vi "DCTMeasure.vi"(1 "Duration Time":refnum<vi>, 2 "Update Time":refnum<vi>, 3 "Time Left":refnum<vi>, 7 "Detectors Select":enum32{"4 Detectors", "8 Detectors"}(ring), 12 "Detector Buttons":refnum<vi>, 13 "Detector Indicators":refnum<vi>, 14 "g2":refnum<vi>) -> (6 "Intensity data":string, 8 "tau data":string, 10 "g2 data":string)   [LabVIEW 2011]
uses:
  DCS/flex05-4chPascal.dll
  DCS/flex05oem8chautoPASCAL.dll
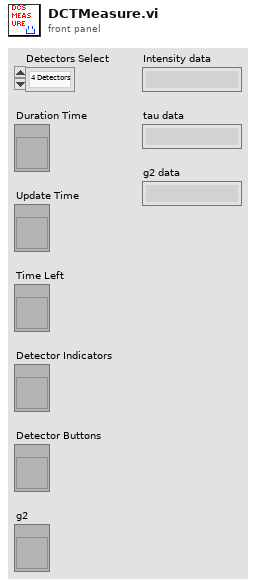
[diagram p1: front panel]
types:
  T1 = cluster{"btnDet 1":bool, "btnDet 2":bool, "btnDet 3":bool, "btnDet 4":bool, "btnDet 5":bool, "btnDet 6":bool, "btnDet 7":bool, "btnDet 8":bool}
  T2 = cluster{"Intensity Array[0]":sgl, "Intensity Array[1]":sgl, "Intensity Array[2]":sgl, "Intensity Array[3]":sgl, "Intensity Array[4]":sgl, "Intensity Array[5]":sgl, "Intensity Array[6]":sgl, "Intensity Array[7]":sgl}
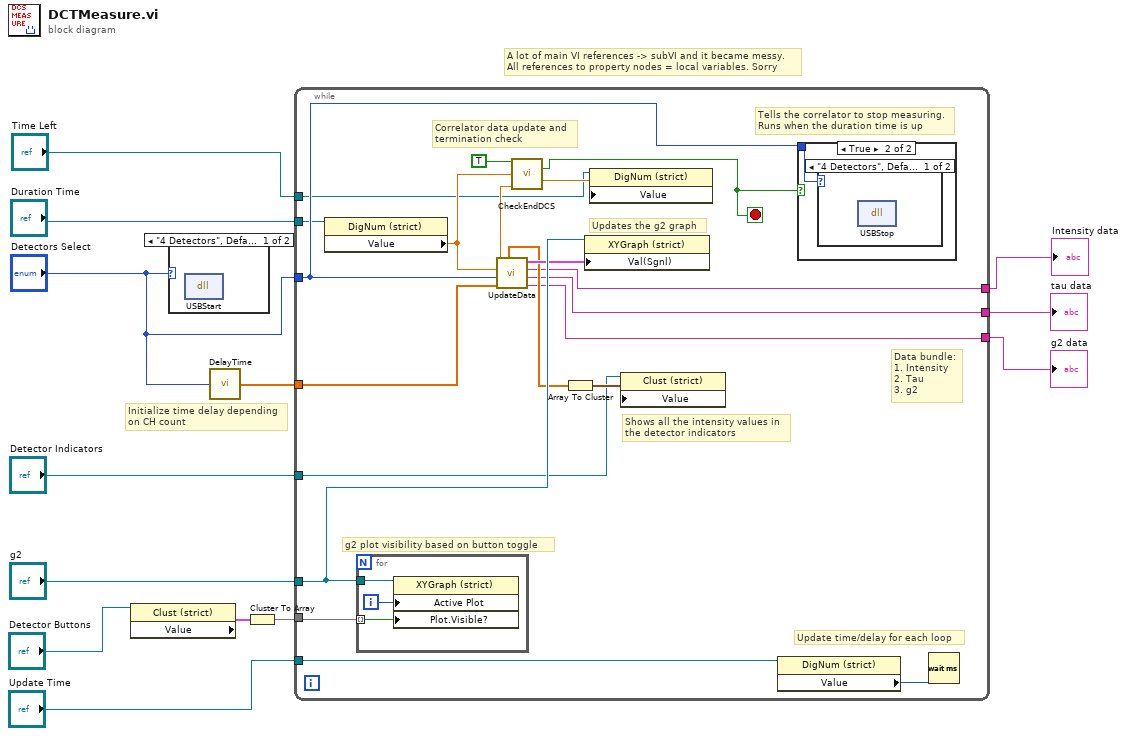
[diagram p0: block diagram]
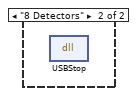
[diagram p3: hidden frame]
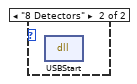
[diagram p4: hidden frame]
diagram:
  # "A lot of main VI references -> subVI and it became messy.\nAll references to property nodes = local variables. Sorry"
  # "Initialize time delay depending\non CH count"
  n1 = property class="Clust (strict)"(reference="Detector Buttons") -> ("Value"=w7:T1)  [unwired: 1 in, 2 out]
  n2 = case shown="\"4 Detectors\", Default" "Detectors Select" {
    frame "4 Detectors", Default {
      n3 = dll-call lib="C:/LABVIEWcodesWorksInC/UnderDeveopmentNeedChecking/Vincent2017/Dependencies/DCS/flex05-4chPascal.dll" fn="USBStart" label="CH4: USBStart"() -> ()  [unwired: 4 in, 2 out]
    }
    frame "8 Detectors" {
      n4 = dll-call lib="C:/LABVIEWcodesWorksInC/UnderDeveopmentNeedChecking/Vincent2017/Dependencies/DCS/flex05oem8chautoPASCAL.dll" fn="USBStart" label="CH8: USBStart"() -> ()  [unwired: 4 in, 2 out]
    }
  }
  n5 = call "DelayTime.vi"("Detector Select"="Detectors Select") -> ("Delaytime"=w6:sgl[])
  n6 = Cluster To Array(cluster=w7) -> (array=w8:bool[])
  n7 = while {
    tunnel: "Detectors Select" -> [w18]
    tunnel: w6 -> [w25]
    tunnel: w8 -> [w33]
    tunnel: "g2" -> [w27]
    tunnel: [w21] -> w11
    tunnel: [w20] -> w12
    tunnel: [w19] -> w13
    tunnel: "Update Time" -> [w17]
    tunnel: "Duration Time" -> [w16]
    tunnel: "Time Left" -> [w15]
    tunnel: "Detector Indicators" -> [w14]
    stop <- w22 stop-if-true
    # "Data bundle:\n1. Intensity\n2. Tau\n3. g2"
    # "Correlator data update and\ntermination check"
    # "Updates the g2 graph"
    # "Shows all the intensity values in\nthe detector indicators"
    # "Update time/delay for each loop"
    # "g2 plot visibility based on button toggle"
    # "Tells the correlator to stop measuring.\nRuns when the duration time is up"
    n8 = property class="DigNum (strict)"(reference=w16) -> ("Value"=w31:sgl)  [unwired: 1 in, 2 out]
    n9 = for {
      tunnel: w33 -> [w36] mode=indexing
      tunnel: w27 -> [w37]
      i -> [w35]
      n10 = property on="Property Node" class="XYGraph (strict)"(reference=w37, "Active Plot"=w35, "Plot.Visible?"=w36) -> ()  [unwired: 1 in, 2 out]
    }
    n11 = call "UpdateData.vi"("Delay Time"=w25, "Detector Select"=w18, "Duration Time (ms)"=w31) -> ("g2 data"=w19:string, "tau data"=w20:string, "Intensity data"=w21:string, "g2 Display"=w26:cluster{"Delay Time":sgl[], sgl[]}[], "Intensity Array"=w23:sgl[], "Elapsed Time(s)"=w28:sgl)  [unwired: 1 out]
    n12 = call "CheckEndDCS.vi"("start"=TRUE, "duration time"=w31, "elapsed time"=w28) -> ("stopped"=w22:bool, "time left"=w30:sgl)  [unwired: 11 in]
    n13 = Array To Cluster(array=w23) -> (cluster=w24:T2)
    n14 = property class="XYGraph (strict)"(reference=w27, "Val(Sgnl)"=w26) -> ()  [unwired: 1 in, 2 out]
    n15 = property class="DigNum (strict)"(reference=w15, "Value"=w30) -> ()  [unwired: 1 in, 2 out]
    n16 = property class="Clust (strict)"(reference=w14, "Value"=w24) -> ()  [unwired: 1 in, 2 out]
    n17 = property class="DigNum (strict)"(reference=w17) -> ("Value"=w32:u32)  [unwired: 1 in, 2 out]
    n18 = case shown="True" w22 {
      tunnel: w18 -> [_ w34]
      frame False {
      }
      frame True {
        n19 = case shown="\"4 Detectors\", Default" w34 {
          frame "4 Detectors", Default {
            n20 = dll-call lib="C:/LABVIEWcodesWorksInC/UnderDeveopmentNeedChecking/Vincent2017/Dependencies/DCS/flex05-4chPascal.dll" fn="USBStop" label="CH4: USBStop"() -> ()  [unwired: 4 in, 2 out]
          }
          frame "8 Detectors" {
            n21 = dll-call lib="C:/LABVIEWcodesWorksInC/UnderDeveopmentNeedChecking/Vincent2017/Dependencies/DCS/flex05oem8chautoPASCAL.dll" fn="USBStop" label="CH8: USBStop"() -> ()  [unwired: 4 in, 2 out]
          }
        }
      }
    }
    n22 = Wait (ms)(milliseconds to wait=w32) -> ()  [unwired: 1 out]
  }
  "g2 data" <- w13
  "tau data" <- w12
  "Intensity data" <- w11
